vi "Read Part Beads.vi"() -> ()   [LabVIEW 2016]
panel:
  out "Numeric":i32
  out "Current Layer":T1
  in  "Layer Data":T2(array[cluster])
  in  "file path (dialog if empty)":path
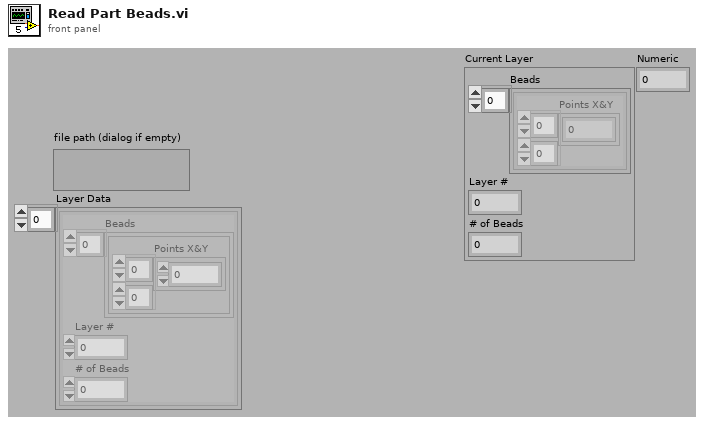
[diagram p1: front panel]
types:
  T1 = cluster{"Beads":cluster{"Points X&Y":dbl[][]}[], "Layer #":dbl, "# of Beads":dbl}
  T2 = cluster{"Beads":cluster{"Points X&Y":dbl[][]}[], "Layer #":dbl, "# of Beads":dbl}[]
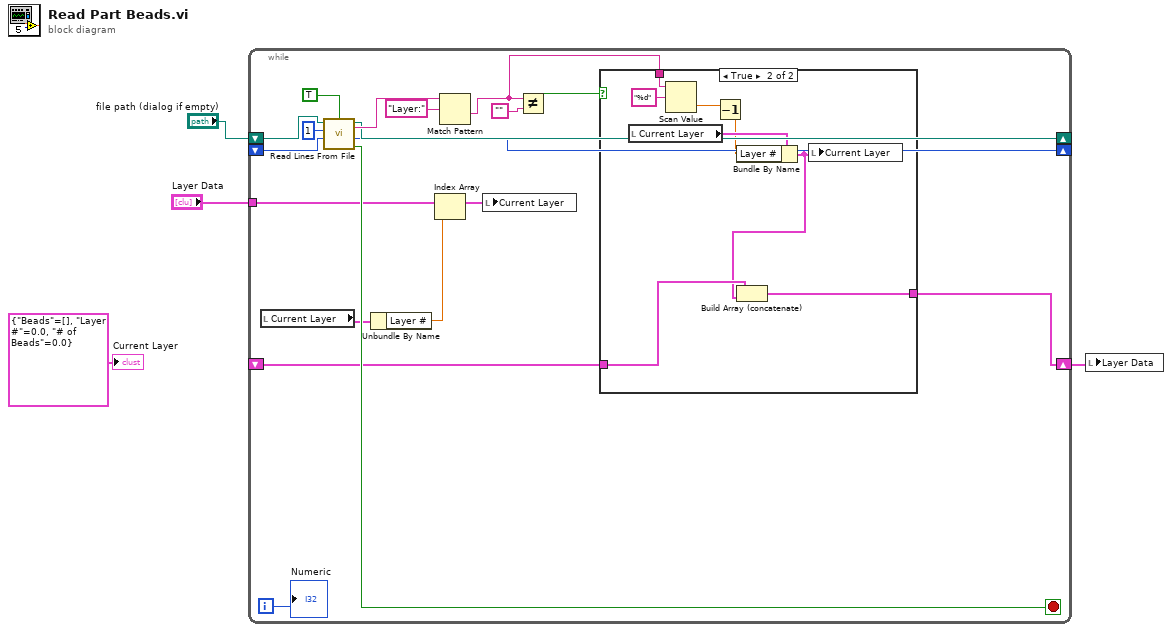
[diagram p0: block diagram]
diagram:
  n1 = while {
    shift-right: [w18] -> _
    shift-left: "file path (dialog if empty)" -> [w23]
    shift-right: [w16] -> _
    shift-left: _ -> [w15]
    tunnel: "Layer Data" -> [w14]
    shift-right: [w6] -> w1
    shift-left: _ -> [w5]
    i -> [w8]
    stop <- w22 stop-if-true
    n2 = local read "Current Layer"() -> (w10:T1)
    n3 = call <vilib>:"Read Lines From File.vi"("convert eol? (no:F)"=TRUE, "file path (dialog if empty)"=w23, "number of lines (all:-1)"=1, "start of read offset (chars.:0)"=w15) -> ("new file path (Not A Path if cancelled)"=w18:path, "line string"=w20:string, "mark after read (chars.)"=w16:i32, "EOF?"=w22:bool)  [unwired: 2 in]
    n4 = Unbundle By Name(w10) -> ("Layer #"=w9:dbl)
    n5 = Index Array(array=w14, index=w9) -> (element=w7:T1)
    n6 = Match Pattern(string=w20, regular expression="Layer:") -> (after substring=w11:string)  [unwired: 1 in, 3 out]
    n7 = local write "Current Layer"(w7) -> ()
    n8 = Not Equal?(x=w11, y="") -> (x != y?=w12:bool)
    n9 = case shown="True" w12 {
      tunnel: w11 -> [_ w31]
      tunnel: [w24 w27] -> w6
      tunnel: w5 -> [w24 w26]
      frame False {
      }
      frame True {
        n10 = local read "Current Layer"() -> (w30:T1)
        n11 = Scan Value(string=w31, format string="%d") -> (value=w29:dbl)  [unwired: 1 in, 1 out]
        n12 = Decrement(x=w29) -> (x-1=w28:dbl)
        n13 = Bundle By Name(cluster=w30, "Layer #"=w28) -> (w25:T1)
        n14 = Build Array (concatenate)(w26, w25) -> (w27:T2)
        n15 = local write "Current Layer"(w25) -> ()
      }
    }
    "Numeric" <- w8
  }
  n16 = local write "Layer Data"(w1) -> ()
  "Current Layer" <- T1 {"Beads"=[], "Layer #"=0.0, "# of Beads"=0.0} ("element")
